vi "Stitching-Load and sort coordinates_.vi"(9 "Selected rows":i32[](array[numeric]), 10 "Experiment folder names column to use":i32) -> ()   [LabVIEW 2017]
uses:
  Coordinates list window/Globals/Coord window-Globals.vi
  <userlib>/My Palettes.lib/Files & paths/Spreadsheet/Read From Spreadsheet File (string)-Mod.vi
  <userlib>/_OpenG.lib/array/array.llb/Reorder 2D Array2 (String)__ogtk.vi
  <userlib>/_OpenG.lib/array/array.llb/Index 1D Array Elements (String)__ogtk.vi
panel:
  out "Selected row indexes in sorted data":i32[](array[numeric])
  out "Selected rows from sorted data":string[][](array[string])
  out "Sorted Pointers":i32[](array[numeric])
  out "Sorted by Y first, then by X":string[][](array[string])
  out "Original data":string[][](array[string])
  # "X"
  # "Y"
  # "X"
  # "Y"
  # "X"
  # "Y"
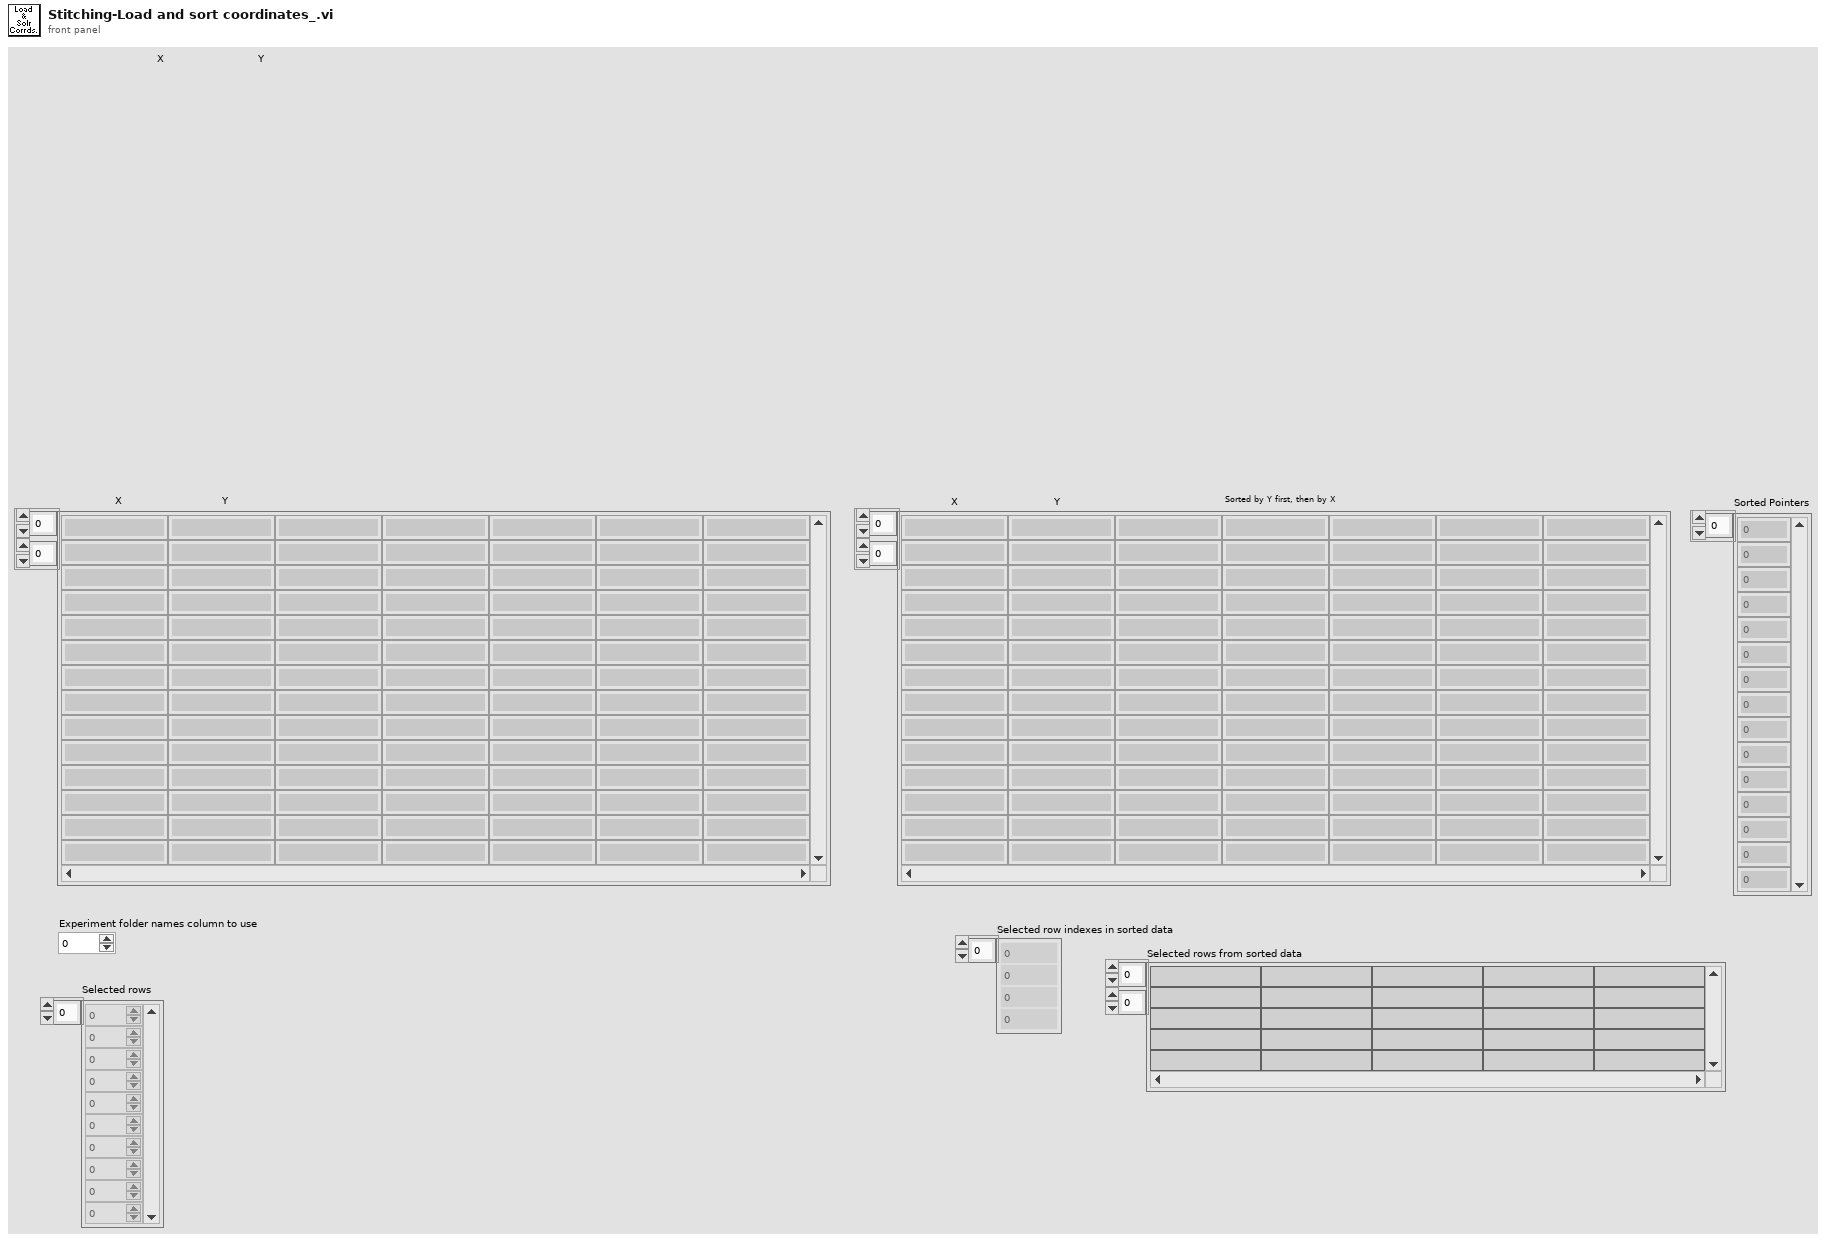
[diagram p1: front panel]
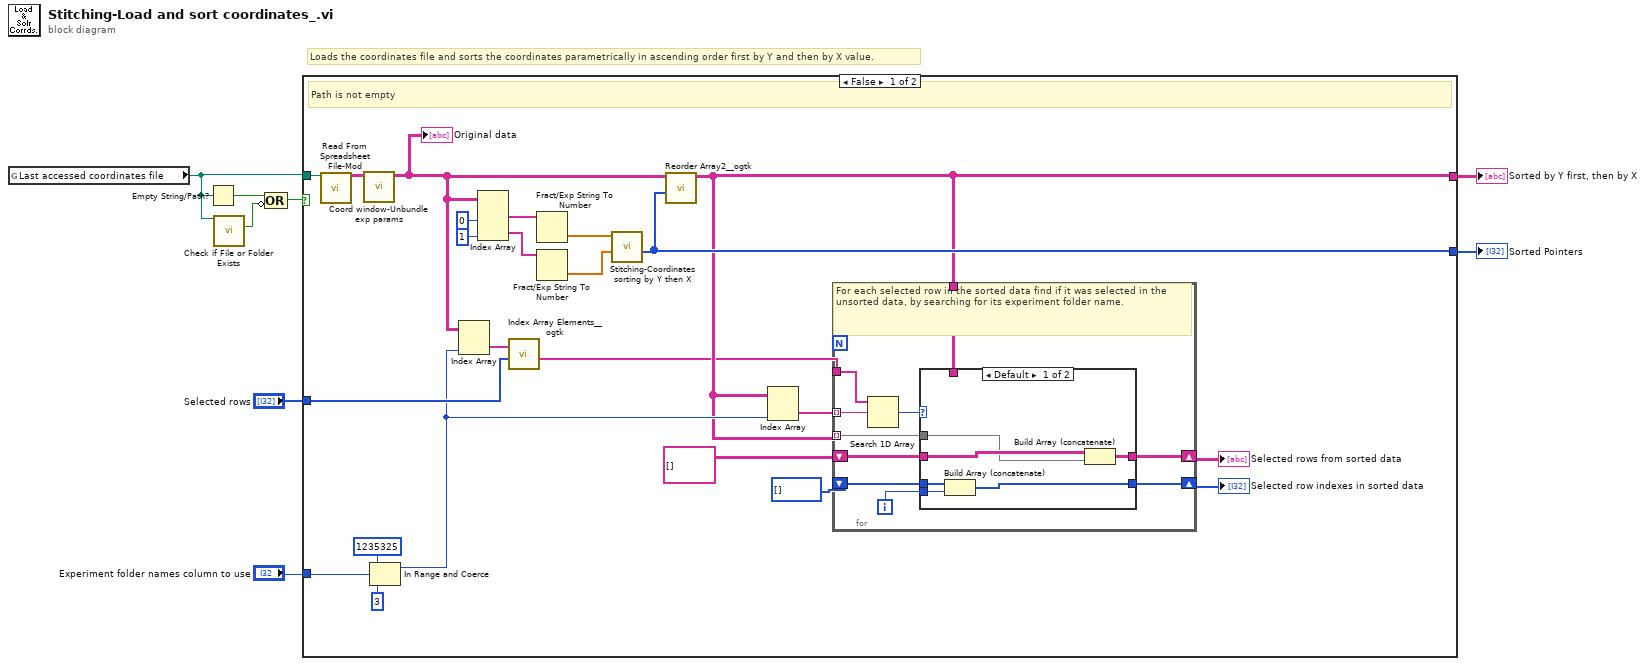
[diagram p0: block diagram]
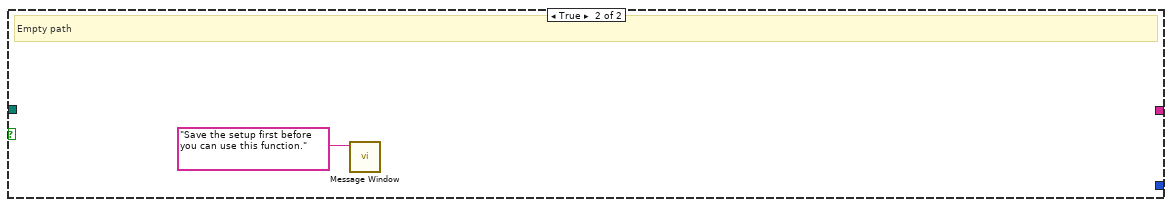
[diagram p3: hidden frame]
diagram:
  # "Loads the coordinates file and sorts the coordinates parametrically in ascending order first by Y and then by X value."
  n1 = global read "Coord window-Globals.vi" "Last accessed coordinates file"() -> (w7:path)
  n2 = Empty String/Path?(string/path=w7) -> (empty?=w5:bool)
  n3 = call <vilib>:"Check if File or Folder Exists.vi"("path"=w7) -> ("file or folder exists?"=w6:bool)  [unwired: 8 in, 2 out]
  n4 = Compound Arithmetic op=OR(w5, invert w6) -> (w4:bool)
  n5 = case shown="False" w4 {
    tunnel: [w23 _] -> w8
    tunnel: w7 -> [w30 _]
    tunnel: [w29 _] -> w3
    tunnel: "Experiment folder names column to use" -> [w27 _]
    tunnel: "Selected rows" -> [w28 _]
    frame False {
      # "Path is not empty"
      n6 = call-poly <userlib>:"Read From Spreadsheet File-Mod.vi"("file path (dialog if empty)"=w30) -> ("all rows"=w31:string[][])  [unwired: 9 in, 5 out]
      n7 = call "Coord window-Unbundle exp params.vi"("Item Names + exp params"=w31) -> ("Item Names"=w22:string[][])  [unwired: 10 in]
      "Original data" <- w22
      n8 = In Range and Coerce(upper limit=1235325, x=w27, lower limit=3) -> (coerced(x)=w24:i32)  [unwired: 1 out]
      n9 = Index Array(array=w22, index (col)=w24) -> (element=w16:string[])  [unwired: 1 in]
      n10 = Index Array(array=w22, index (col) #1=0 ("disabled index (col)"), index (col) #2=1 ("index (col)")) -> (element #1=w19:string[], element #2=w9:string[])  [unwired: 2 in]
      n11 = call-poly <userlib>:"Index Array Elements__ogtk.vi"("indices"=w28, "array"=w16) -> ("elements"=w14:string[])  [unwired: 9 in]
      n12 = Fract/Exp String To Number(string=w19) -> (number=w18:dbl[])  [unwired: 3 in, 1 out]
      n13 = Fract/Exp String To Number(string=w9) -> (number=w17:dbl[])  [unwired: 3 in, 1 out]
      n14 = call "Stitching-Coordinates sorting by Y then X.vi"("Y"=w17, "X"=w18) -> ("Sorted Pointers"=w29:i32[])  [unwired: 8 in, 1 out]
      n15 = call-poly <userlib>:"Reorder Array2__ogtk.vi"("indices"=w29, "array"=w22) -> ("reordered array"=w23:string[][])  [unwired: 9 in]
      n16 = Index Array(array=w23, index (col)=w24) -> (element=w15:string[])  [unwired: 1 in]
      n17 = for {
        tunnel: w15 -> [w34] mode=indexing
        tunnel: w14 -> [w35]
        shift-right: [w40] -> w10
        shift-left: i32[] [] -> [w39]
        tunnel: w23 -> [w38]
        shift-right: [w37] -> w11
        shift-left: string[][] [] -> [w36]
        tunnel: w23 -> [w32] mode=indexing
        i -> [w33]
        # "For each selected row in the sorted data find if it was selected in the unsorted data, by searching for its experiment folder name."
        n18 = Search 1D Array(1D array=w35, element=w34) -> (index of element=w41:i32)  [unwired: 1 in]
        n19 = case shown="Default" w41 {
          tunnel: [w47 w49] -> w40
          tunnel: w39 -> [w46 w49]
          tunnel: w38 -> [_ _]
          tunnel: [w45 w48] -> w37
          tunnel: w36 -> [w44 w48]
          tunnel: w33 -> [w43 _]
          tunnel: w32 -> [w42 _]
          frame Default {
            n20 = Build Array (concatenate)(w46, w43) -> (w47:i32[])
            n21 = Build Array (concatenate)(w44, w42) -> (w45:string[][])
          }
          frame -1 {
          }
        }
      }
      "Selected rows from sorted data" <- w11
      "Selected row indexes in sorted data" <- w10
    }
    frame True {
      # "Empty path"
      n22 = call "Message Window.vi"("Message string"="Save the setup first before you can use this function.") -> ()  [unwired: 10 in, 1 out]
    }
  }
  "Sorted by Y first, then by X" <- w8
  "Sorted Pointers" <- w3
